vi "Get VI Metadata.vi"(8 "error in":errorcluster, 11 "VI ref in":refnum<vi>) -> (0 "error out":errorcluster, 2 "Metadata":T1, 3 "VI ref out":refnum<vi>)   [LabVIEW 2019]
doc: "Get information about the VI and creates an HTML content to be used in the main viewer."
uses:
  Typedefs/VI Metadata.ctl
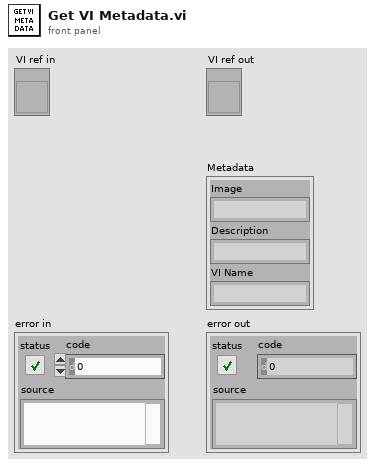
[diagram p1: front panel]
types:
  T1 = typedef "VI Metadata.ctl" = cluster{"Image":string, "Description":string, "VI Name":string}
  T2 = enum32{"invalid VI type", "Standard VI", "Control VI", "Global VI", "Polymorphic VI", "Configuration VI", "SubSystem", "Facade VI", "Method VI", "Statechart Diagram VI"}
  T3 = typedef "imagedata.ctl" = cluster{"image type":i32, "image depth":i32, "image":u8[], "mask":u8[], "colors":u32[], "Rectangle":cluster{"left":i16, "top":i16, "right":i16, "bottom":i16}}
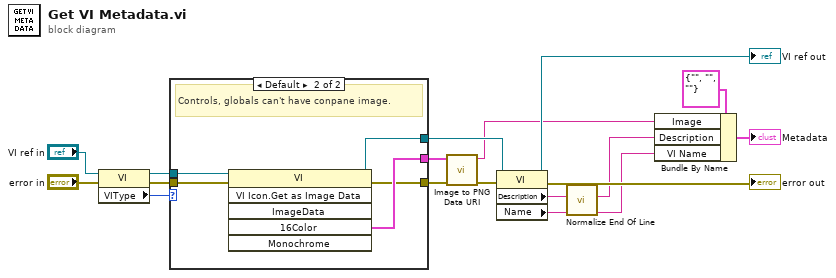
[diagram p0: block diagram]
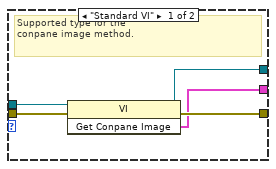
[diagram p2: hidden frame]
diagram:
  n1 = property class="VI"(reference="VI ref in", error in="error in") -> (reference out=w13:refnum<vi>, error out=w15:errorcluster, "VIType"=w14:T2)
  n2 = case shown="Default" w14 {
    tunnel: w15 -> [w22 w23]
    tunnel: [w20 w24] -> w8
    tunnel: w13 -> [w21 w26]
    tunnel: [w19 w25] -> w12
    tunnel: [w18 w27] -> w10
    frame "Standard VI" {
      # "Supported type for the \nconpane image method."
      n3 = invoke class="VI" method="Get Conpane Image"(reference=w21, error in=w22) -> (reference out=w19:refnum<vi>, error out=w20:errorcluster, "Get Conpane Image"=w18:T3)  [unwired: 1 in]
    }
    frame Default {
      # "Controls, globals can't have conpane image."
      n4 = invoke class="VI" method="VI Icon.Get as Image Data"(reference=w26, error in=w23) -> (reference out=w25:refnum<vi>, error out=w24:errorcluster, "16Color"=w27:T3)  [unwired: 4 in, 3 out]
    }
  }
  n5 = call "Image to PNG Data URI.vi"("error in (no error)"=w8, "Image data"=w10) -> ("error out"=w7:errorcluster, "Base64 encoded"=w9:string)  [unwired: 7 in, 1 out]
  n6 = property class="VI"(reference=w12, error in=w7) -> (reference out=→"VI ref out":refnum<vi>, error out=→"error out":errorcluster, "Description"=w4:string, "Name"=w5:string)
  n7 = call <vilib>:"Normalize End Of Line.vi"("string in"=w4) -> ("string out"=w3:string)  [unwired: 7 in]
  n8 = Bundle By Name(cluster=T1 {"Image"="", "Description"="", "VI Name"=""} ("Metadata"), "Image"=w9, "Description"=w3, "VI Name"=w5) -> (→"Metadata":T1)
